vi "CalculateVelAtPoints.vi"(8 "MaxVels":dbl[](array[numeric]), 9 "MaxVel":dbl, 10 "MaxAccel":dbl, 11 "DistancesToEnd":dbl[](array[numeric])) -> (3 "Vel":dbl[](array[numeric]))   [LabVIEW 2017]
panel:
  out "Waveform Graph":dbl[](graph)
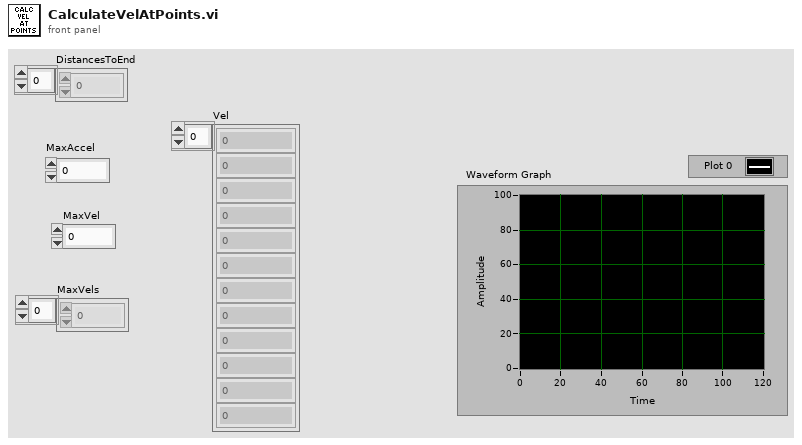
[diagram p1: front panel]
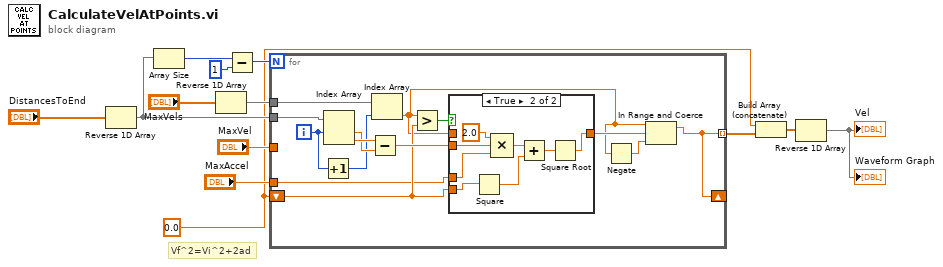
[diagram p0: block diagram]
diagram:
  w3 = 0.0 ("MaxAccel")
  # "Vf^2=Vi^2+2ad"
  n1 = Reverse 1D Array(array="DistancesToEnd") -> (reversed array=w6:dbl[])
  n2 = Array Size(array=w6) -> (size(s)=w13:i32)
  n3 = Reverse 1D Array(array="MaxVels") -> (reversed array=w5:dbl[])
  n4 = Subtract(x=w13, y=1) -> (x-y=w11:i32)
  n5 = for {
    N: w11 -> [_]
    tunnel: w6 -> [w27]
    shift-right: [w16] -> _
    shift-left: w3 -> [w19]
    tunnel: "MaxAccel" -> [w18]
    tunnel: "MaxVel" -> [_]
    tunnel: w5 -> [w24]
    tunnel: [w16] -> w4 mode=indexing
    i -> [w23]
    n6 = Increment(x=w23) -> (x+1=w22:i32)
    n7 = Index Array(array=w27, index #1=w23) -> (element #1=w25:dbl, element #2=w26:dbl)  [unwired: 1 in]
    n8 = Subtract(x=w26, y=w25) -> (x-y=w20:dbl)
    n9 = Index Array(array=w24, index=w22) -> (element=w14:dbl)
    n10 = Greater?(x=w14, y=w19) -> (0:w21:bool)
    n11 = case shown="True" w21 {
      tunnel: w20 -> [_ w34]
      tunnel: [w28 w29] -> w17
      tunnel: w19 -> [_ w36]
      tunnel: w14 -> [w28 _]
      tunnel: w18 -> [_ w33]
      frame False {
      }
      frame True {
        n12 = Square(x=w36) -> (x^2=w32:dbl)
        n13 = Compound Arithmetic op=MULTIPLY(2.0 ("value"), w34, w33) -> (w31:dbl)
        n14 = Add(x=w31, y=w32) -> (x+y=w30:dbl)
        n15 = Square Root(x=w30) -> (sqrt(x)=w29:dbl)
      }
    }
    n16 = Negate(x=w14) -> (-x=w15:dbl)
    n17 = In Range and Coerce(upper limit=w14, x=w17, lower limit=w15) -> (coerced(x)=w16:dbl)  [unwired: 1 out]
  }
  n18 = Build Array (concatenate)(w3, w4) -> (w2:dbl[])
  n19 = Reverse 1D Array(array=w2) -> (reversed array=→"Vel" →"Waveform Graph":dbl[])
